vi "Translate_TABLE.vi"(8 "error IN":errorcluster, 10 "Cle":string, 11 "Tbl Refnum":refnum<vi>) -> (0 "error out":errorcluster)   [LabVIEW 2011]
uses:
  Dictionnary/EnumCommandDictionnaire.ctl
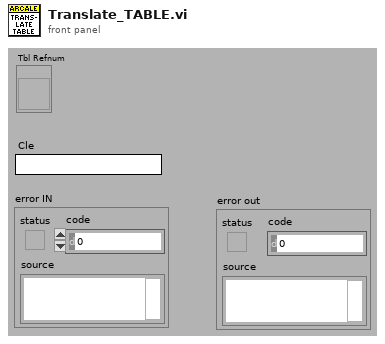
[diagram p1: front panel]
types:
  T1 = typedef "EnumCommandDictionnaire.ctl" = enum16{"Load", "Translate", "Save", "GetDico", "Set : A traduire = Vrai", "Set : A Traduire = Faux", "SetDico"}
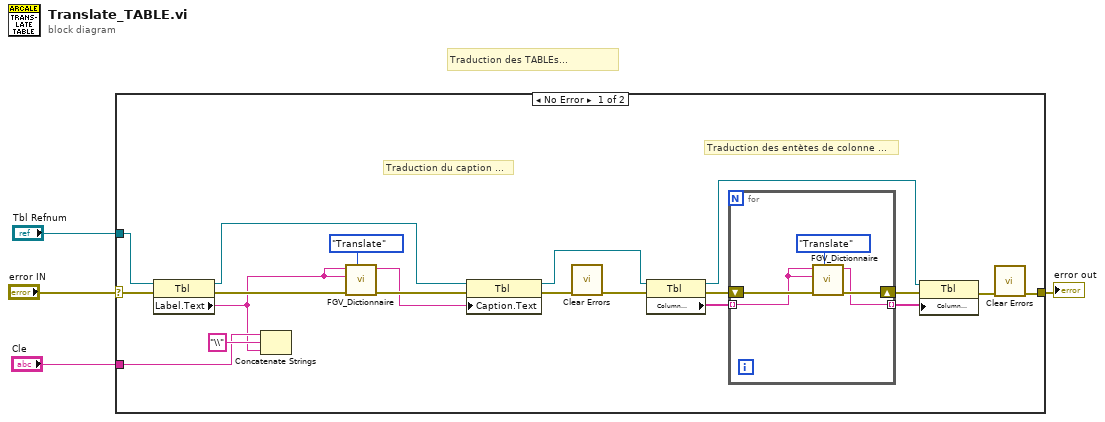
[diagram p0: block diagram]
diagram:
  # "Traduction des TABLEs..."
  n1 = case shown="No Error" "error IN" {
    selector: "error IN" -> [w24 w30]
    tunnel: "Tbl Refnum" -> [w23 _]
    tunnel: "Cle" -> [w19 _]
    tunnel: [w7 w30] -> w1
    frame No Error {
      # "Traduction des entètes de colonne ..."
      # "Traduction du caption ..."
      n2 = property class="Tbl"(reference=w23, error in=w24) -> (reference out=w20:refnum<vi>, error out=w17:errorcluster, "Label.Text"=w14:string)
      n3 = Concatenate Strings(w19, "\\" ("string"), w14) -> ()  [unwired: 1 out]
      n4 = call "FGV_Dictionnaire.vi"("Command"=EnumCommandDictionnaire."Translate", "error in (no error)"=w17, "Chaîne"=w14, "Clé"=w14) -> ("error out"=w16:errorcluster, "Traduction"=w15:string)  [unwired: 5 in, 1 out]
      n5 = property class="Tbl"(reference=w20, error in=w16, "Caption.Text"=w15) -> (reference out=w12:refnum<vi>, error out=w21:errorcluster)
      n6 = call <vilib>:"Clear Errors.vi"("error in (no error)"=w21) -> ("error out"=w13:errorcluster)  [unwired: 6 in]
      n7 = property class="Tbl"(reference=w12, error in=w13) -> (reference out=w5:refnum<vi>, error out=w10:errorcluster, "Column Headers[]"=w11:string[])
      n8 = for {
        tunnel: w11 -> [w26] mode=indexing
        shift-right: [w27] -> w9
        shift-left: w10 -> [w28]
        tunnel: [w25] -> w6 mode=indexing
        n9 = call "FGV_Dictionnaire.vi"("Command"=EnumCommandDictionnaire."Translate", "error in (no error)"=w28, "Chaîne"=w26, "Clé"=w26) -> ("error out"=w27:errorcluster, "Traduction"=w25:string)  [unwired: 5 in, 1 out]
      }
      n10 = property class="Tbl"(reference=w5, error in=w9, "Column Headers[]"=w6) -> (error out=w8:errorcluster)  [unwired: 1 out]
      n11 = call <vilib>:"Clear Errors.vi"("error in (no error)"=w8) -> ("error out"=w7:errorcluster)  [unwired: 6 in]
    }
    frame Error {
    }
  }
  "error out" <- w1
